vi "Spin Move.vi"(10 "Motor In":cluster{"Port":T1, "Port":T1}={"Port"=1, "Port"=3} {"Port" items=["Port A", "Port B", "Port C", "Port D"]; "Port" items=["Port A", "Port B", "Port C", "Port D"]}, 11 "Ref In":T2) -> (2 "Motor Out":cluster{"Port":T1, "Port":T1} {"Port" items=["Port A", "Port B", "Port C", "Port D"]; "Port" items=["Port A", "Port B", "Port C", "Port D"]}, 3 "Ref Out":T2)   [LabVIEW 2014]
doc: "Spin Move\n\nIdle/Default State:\n\nContinuously pivot, so that it stays at the center, and so that it can sense front all angles. \nDefensive move if competitor executes the same code, which will at least result in a timed out draw.\n\nBeverly Abadines\nPHY 350\nBAP7"
uses:
  <vilib>/NXT/Subs/LVHSConnector.ctl
  <vilib>/NXT/LegoClasses/BrickReference/BrickReference.lvclass
  <vilib>/NXT/Block Support/NXT_OutputPort.ctl
  <vilib>/NXT/NXTIO Xnodes/NXTIONodeSubVIs/NXTMoveMotors.vi
  <vilib>/NXT/NXTIO Xnodes/AddressXNode/NXTIOAddress.xnode
  <vilib>/NXT/NXTIO Xnodes/NXTIOXNode/NXTIO.xnode
panel:
  # "Beverly Abadines\nPHY 350\nP7"
  # "Spin Move"
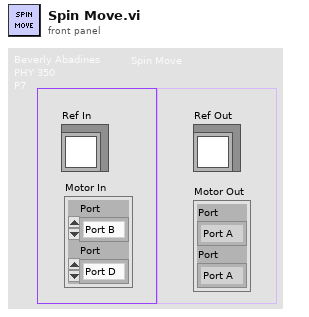
[diagram p1: front panel]
types:
  T1 = typedef "NXT_OutputPort.ctl" = u8
  T2 = typedef "LVHSConnector.ctl" = refnum<class "BrickReference.lvclass">
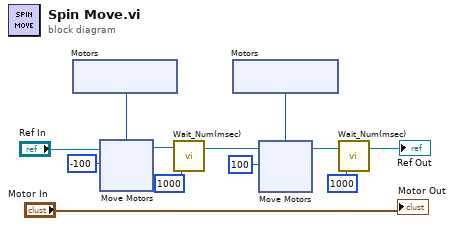
[diagram p0: block diagram]
diagram:
  n1 = xnode "Motors"() -> ("Motor"=w12:T1)
  n2 = xnode "Move Motors"("Power/Speed 1"=i8 -100, "Motors"=w12, "NXT/EV3"="Ref In") -> ("NXT/EV3"=w8:T2)
  n3 = call <vilib>:"Wait_Num(msec).vi"("Time (100 msec)"=u32 1000, "NXT/EV3"=w8) -> ("NXT/EV3"=w7:T2)  [unwired: 2 in]
  n4 = xnode "Motors"() -> ("Motor"=w11:T1)
  n5 = xnode "Move Motors"("Power/Speed 1"=i8 100, "Motors"=w11, "NXT/EV3"=w7) -> ("NXT/EV3"=w6:T2)
  n6 = call <vilib>:"Wait_Num(msec).vi"("Time (100 msec)"=u32 1000, "NXT/EV3"=w6) -> ("NXT/EV3"=→"Ref Out":T2)  [unwired: 2 in]
  "Motor Out" <- "Motor In"
